vi "Footer Correction Dialogue.vi"(8 "Error In":errorcluster, 10 "Footer Image In":T1, 11 "Footer In":string) -> (0 "Error Out":errorcluster, 2 "DateTime Out":timestamp)   [LabVIEW 2018, in "Main.lvlib"]
uses:
  Main.lvlib
  <vilib>/vision/Image Controls.llb/IMAQ Image.ctl
  receipt parsing/Receipt Parsing.lvlib
panel:
  out "Footer":string
  in  "DateTime in Footer Text":timestamp
  in  "OK Button":bool
  out "Footer Image":T1(plugin-control)
  # "Date/time did not parse\nPlease input manually"
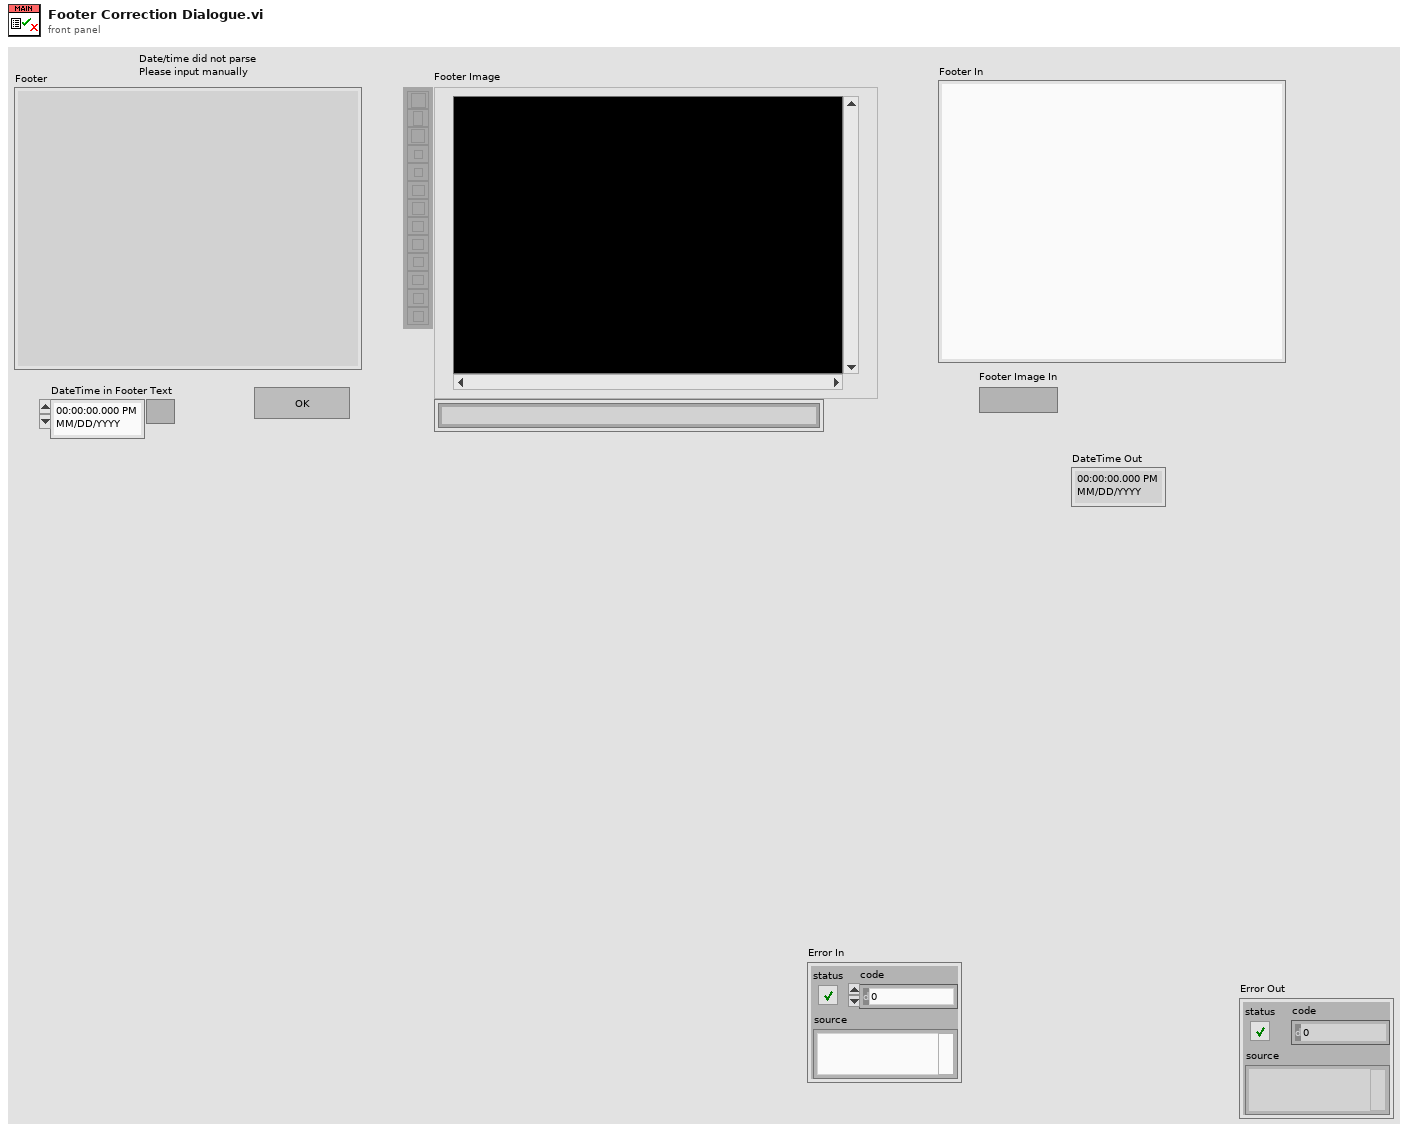
[diagram p1: front panel]
types:
  T1 = typedef "IMAQ Image.ctl" = refnum<image>
  T2 = typedef "LVDateTimeRec.ctl" = cluster{"fractional second":dbl, "second":i32, "minute":i32, "hour":i32, "day of month":i32, "month":i32, "year":i32, "day of week":i32, "day of year":i32, "DST":i32}
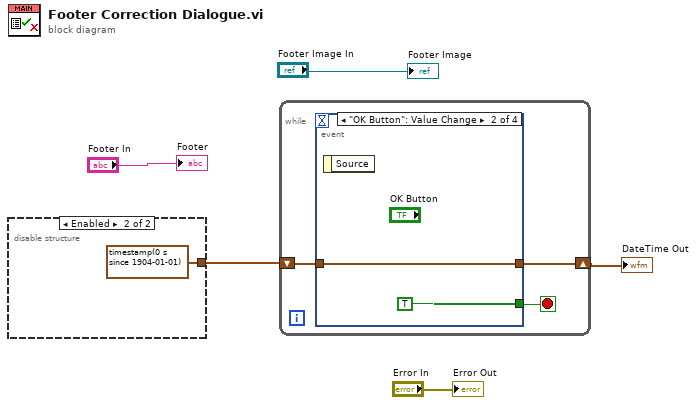
[diagram p0: block diagram]
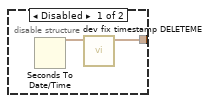
[diagram p2: hidden frame]
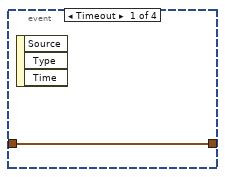
[diagram p3: hidden frame]
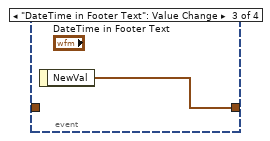
[diagram p4: hidden frame]
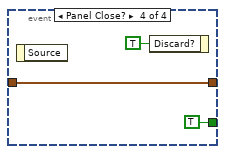
[diagram p5: hidden frame]
diagram:
  n1 = disable-structure shown="Enabled" {
    disable-tunnel: [w7 timestamp(0 s since 1904-01-01) ("time stamp")] -> w3
    frame Disabled {
      n2 = Seconds To Date/Time() -> (time stamp (now)=w6:timestamp, date time rec=w8:T2)  [unwired: 1 in]
      n3 = call "dev fix timestamp DELETEME.vi"("date time rec"=w8) -> ("time stamp"=w7:timestamp)  [unwired: 10 in]
    }
    frame Enabled {
    }
  }
  n4 = while {
    shift-right: [w11] -> w1
    shift-left: w3 -> [w10]
    stop <- w12 stop-if-true
    n5 = event shown="[1] \"OK Button\": Value Change" {
      selector: _ -> [_ _ _ _]
      dyn-events: _ -> [_ _ _ _]
      timeout: _ -> [_ _ _ _]
      tunnel: [_ TRUE _ TRUE] -> w12
      tunnel: [w13 w14 w16 w17] -> w11
      tunnel: w10 -> [w13 w14 _ w17]
      event Timeout {
        n6 = event-data() -> ()  [unwired: 1 in, 3 out]
      }
      event "OK Button": Value Change {
        n7 = event-data() -> ()  [unwired: 1 in, 1 out]
      }
      event "DateTime in Footer Text": Value Change {
        n8 = event-data() -> ("NewVal"=w16:timestamp)  [unwired: 1 in]
      }
      event Panel Close? {
        n9 = event-data() -> ()  [unwired: 1 in, 1 out]
        n10 = event-data("Discard?"=TRUE) -> ()  [unwired: 1 in, 1 out]
      }
    }
  }
  "DateTime Out" <- w1
  "Footer Image" <- "Footer Image In"
  "Error Out" <- "Error In"
  "Footer" <- "Footer In"
